vi "setPublisher.vi"(10 "Publisher":refnum<class "Publisher.lvclass">, 11 "Model in":refnum<class "Model.lvclass">) -> (3 "Model out":refnum<class "Model.lvclass">)   [LabVIEW 2016, in "Model.lvclass"]
uses:
  Model.lvclass
  Publisher/Publisher.lvclass
  Model.lvclass/Model.ctl
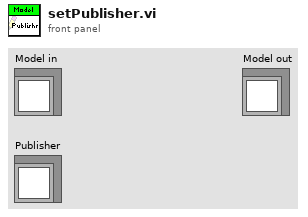
[diagram p1: front panel]
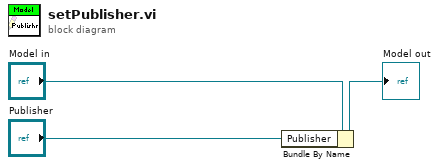
[diagram p0: block diagram]
diagram:
  n1 = Bundle By Name(cluster="Model in", "Publisher"="Publisher") -> (→"Model out":refnum<class "Model.lvclass">)
